vi "Launcher.vi"   [LabVIEW 2020, in "GUI Actor.lvlib" / "GUI Actor.lvclass"]
uses:
  GUI Actor.lvclass
  C:/Program Files (x86)/National Instruments/LabVIEW 2020/vi.lib/ActorFramework/Actor/Actor.lvclass
  <vilib>/ActorFramework/Actor/Actor.lvclass
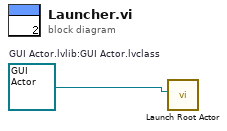
[diagram p0: block diagram]
diagram:
  w1 = refnum<class "GUI Actor.lvclass"> refnum  # GUI Actor.lvlib:GUI Actor.lvclass
  n1 = call <vilib>:"Launch Root Actor.vi"("Actor"=w1) -> ()  [unwired: 9 in, 2 out]
